vi "calculate tiling positions.vi"(7 "Single Plane?":bool, 8 "error in (no error)":errorcluster, 9 "overlap percentage":dbl) -> (0 "error out 2":errorcluster, 2 "Array 2 - for Zstack tiling use this":dbl[][][](array[numeric]), 3 "2D Array for single plane tiling or Slow Z Tiling":dbl[][](array[numeric]))   [LabVIEW 2012]
doc: "SciScan 1.2 160622"
uses:
  GFG/GFGnumericGet.vi
  GFG/GFGbooleanGet.vi
  GFG/GFG library.lvlib
panel:
  out "Array":dbl[][](array[numeric])
  out "error out":errorcluster
  out "data":dbl[][](array[numeric])
  out "3D Array for Standard Z Tiling":dbl[][][](array[numeric])
  in  "no of frames per tile":dbl
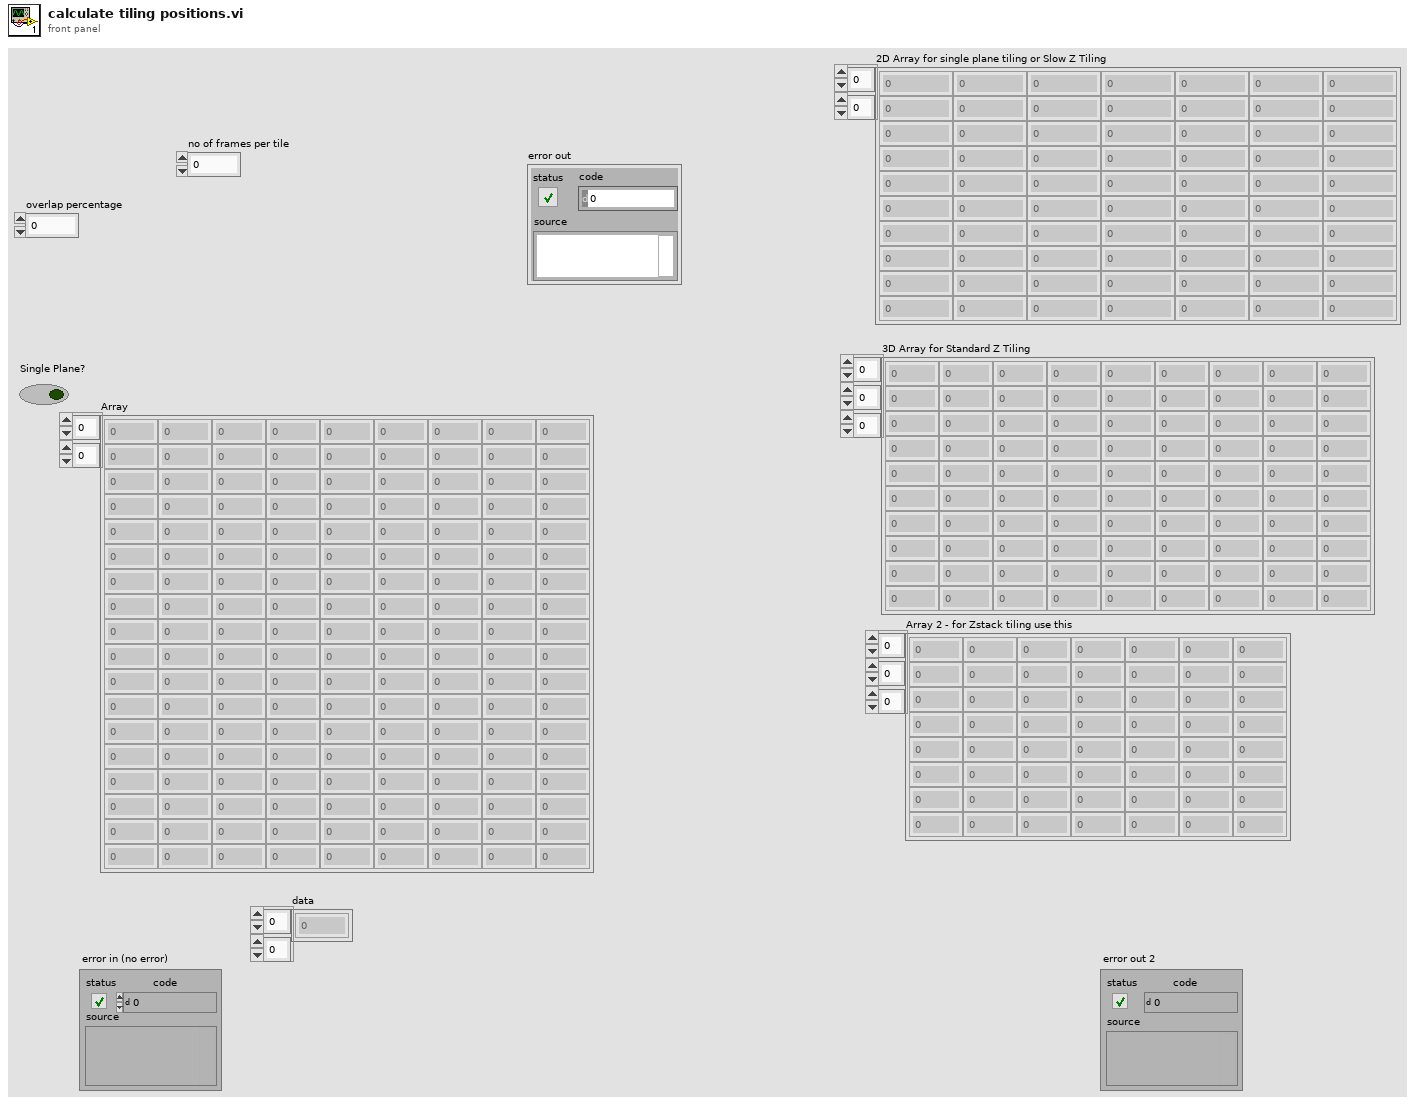
[diagram p1: front panel]
types:
  T1 = cluster{"moveXabs":dbl, "moveYabs":dbl, "moveZabs":dbl}
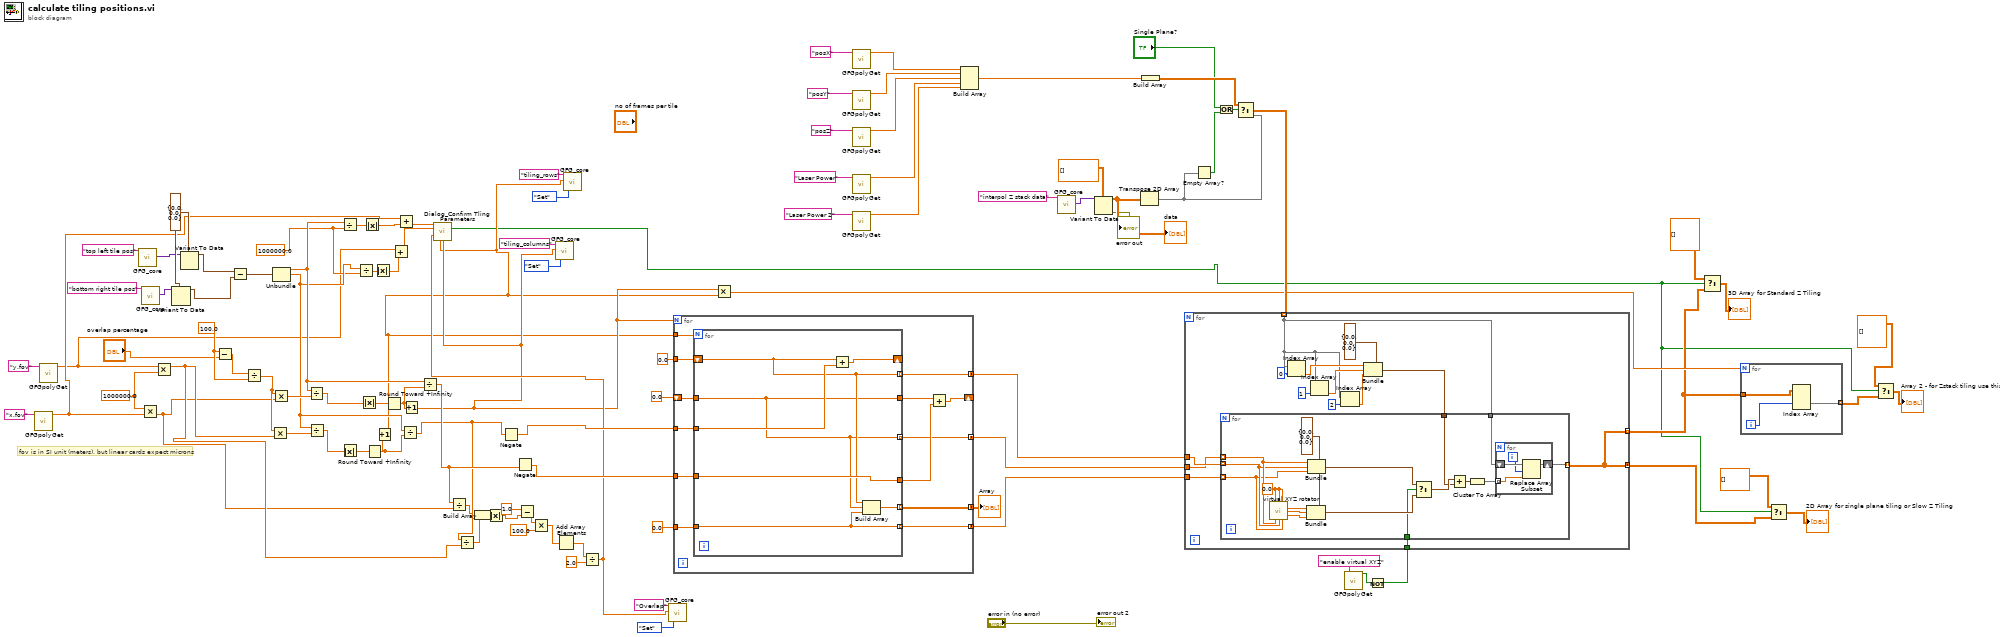
[diagram p0: block diagram]
diagram:
  w22 = 1000000.0 ("y")
  w51 = 1000000.0 ("y")
  w67 = cluster{"rel x":dbl, "rel y":dbl, "rel z":dbl} {"rel x"=0.0, "rel y"=0.0, "rel z"=0.0} ("top left")
  w55 = 100.0 ("x")
  # "fov is in SI unit (meters), but linear cards expect microns"
  n1 = call-poly "GFGpolyGet.vi"("Variable Name in"="x.fov") -> ("Numeric"=w4:dbl)  [unwired: 8 in, 2 out]
  n2 = call-poly "GFGpolyGet.vi"("Variable Name in"="y.fov") -> ("Numeric"=w3:dbl)  [unwired: 8 in, 2 out]
  n3 = call "GFG_core.vi"("Variable Name in"="top left tile pos") -> ("Variant Out"=w63:variant)  [unwired: 12 in, 6 out]
  n4 = call "GFG_core.vi"("Variable Name in"="bottom right tile pos") -> ("Variant Out"=w65:variant)  [unwired: 12 in, 6 out]
  n5 = Multiply(x=w51, y=w4) -> (x*y=w26:dbl)
  n6 = Multiply(x=w3, y=w51) -> (x*y=w27:dbl)
  n7 = Variant To Data(type=w67, Variant=w65) -> (data=w66:cluster{"rel x":dbl, "rel y":dbl, "rel z":dbl})  [unwired: 1 in, 1 out]
  n8 = Variant To Data(type=w67, Variant=w63) -> (data=w64:cluster{"rel x":dbl, "rel y":dbl, "rel z":dbl})  [unwired: 1 in, 1 out]
  n9 = Subtract(x=w55, y="overlap percentage") -> (x-y=w54:dbl)
  n10 = Subtract(x=w64, y=w66) -> (x-y=w53:cluster{"rel x":dbl, "rel y":dbl, "rel z":dbl})
  n11 = Divide(x=w54, y=w55) -> (x/y=w50:dbl)
  n12 = Multiply(x=w50, y=w27) -> (x*y=w56:dbl)
  n13 = Unbundle(w53) -> ("rel x"=w24:dbl, "rel y"=w23:dbl)  [unwired: 1 out]
  n14 = Multiply(x=w50, y=w26) -> (x*y=w57:dbl)
  n15 = Divide(x=w24, y=w57) -> (x/y=w60:dbl)
  n16 = Divide(x=w23, y=w56) -> (x/y=w49:dbl)
  n17 = Divide(x=w24, y=w22) -> (x/y=w21:dbl)
  n18 = Absolute Value(x=w49) -> (abs(x)=w58:dbl)
  n19 = Divide(x=w23, y=w22) -> (x/y=w20:dbl)
  n20 = Absolute Value(x=w60) -> (abs(x)=w59:dbl)
  n21 = Absolute Value(x=w21) -> (abs(x)=w2:dbl)
  n22 = Round Toward +Infinity(x=w58) -> (ceil(x): smallest int >= x=w43:dbl)
  n23 = Absolute Value(x=w20) -> (abs(x)=w1:dbl)
  n24 = Increment(x=w43) -> (x+1=w17:dbl)
  n25 = Round Toward +Infinity(x=w59) -> (ceil(x): smallest int >= x=w44:dbl)
  n26 = Add(x=w3, y=w1) -> (x+y=w5:dbl)
  n27 = Add(x=w4, y=w2) -> (x+y=w6:dbl)
  n28 = Divide(x=w23, y=w43) -> (x/y=w37:dbl)
  n29 = Increment(x=w44) -> (x+1=w18:dbl)
  n30 = Divide(x=w24, y=w44) -> (x/y=w38:dbl)
  n31 = Divide(x=w38, y=w26) -> (x/y=w36:dbl)
  n32 = Divide(x=w37, y=w27) -> (x/y=w35:dbl)
  n33 = Build Array(w36, w35) -> (w33:dbl[])
  n34 = Absolute Value(x=w33) -> (abs(x)=w25:dbl[])
  n35 = Negate(x=w37) -> (-x=w42:dbl)
  n36 = Negate(x=w38) -> (-x=w41:dbl)
  n37 = Subtract(x=1.0, y=w25) -> (x-y=w32:dbl[])
  n38 = Multiply(x=w32, y=100.0 ("x")) -> (x*y=w30:dbl[])
  n39 = call "GFG_core.vi"("Variable Name in"="tiling_columns", "Variant in"=w18, "Action"=enum16{"Init", "Set", "Get", "Clear"}."Set") -> ()  [unwired: 10 in, 7 out]
  n40 = Add Array Elements(numeric array=w30) -> (sum=w29:dbl)
  n41 = call "GFG_core.vi"("Variable Name in"="tiling_rows", "Variant in"=w17, "Action"=enum16{"Init", "Set", "Get", "Clear"}."Set") -> ()  [unwired: 10 in, 7 out]
  n42 = Divide(x=w29, y=2.0) -> (x/y=w19:dbl)
  n43 = call "Dialog_Confirm Tling Parameters.vi"("x FOV"=w6, "y FOV"=w5, "actual \noverlap\npercentage"=w19, "Tiling Rows"=w17, "Tiling Columns"=w18) -> ("Cancelled?"=w7:bool)  [unwired: 9 in, 1 out]
  n44 = call "GFG_core.vi"("Variable Name in"="Overlap", "Variant in"=w19, "Action"=enum16{"Init", "Set", "Get", "Clear"}."Set") -> ()  [unwired: 10 in, 7 out]
  n45 = for {
    N: w18 -> [_]
    shift-right: [w113] -> _
    shift-left: 0.0 ("Numeric") -> [w115]
    tunnel: w42 -> [w112]
    tunnel: [w111] -> w98 mode=concatenating
    tunnel: w41 -> [w109]
    tunnel: [w108] -> w97 mode=concatenating
    tunnel: [w107] -> w96 mode=concatenating
    tunnel: w17 -> [w106]
    tunnel: 0.0 ("Numeric") -> [w116]
    tunnel: 0.0 ("Numeric") -> [w105]
    tunnel: [w104] -> w73 mode=concatenating
    n46 = for {
      N: w106 -> [_]
      shift-right: [w122] -> _
      shift-left: w116 -> [w120]
      tunnel: w112 -> [w123]
      tunnel: [w120] -> w111 mode=indexing
      tunnel: [w121] -> w110
      tunnel: w109 -> [w121]
      tunnel: [w119] -> w108 mode=indexing
      tunnel: w105 -> [w118]
      tunnel: [w118] -> w107 mode=indexing
      tunnel: w115 -> [w119]
      tunnel: [w119] -> w114
      tunnel: [w117] -> w104 mode=indexing
      n47 = Add(x=w120, y=w123) -> (x+y=w122:dbl)
      n48 = Build Array(w120, w119, w118) -> (w117:dbl[])
    }
    n49 = Add(x=w114, y=w110) -> (x+y=w113:dbl)
  }
  "Array" <- w73
  n50 = Multiply(x=w18, y=w17) -> (x*y=w72:dbl)
  n51 = call-poly "GFGpolyGet.vi"("Variable Name in"="posX") -> ("Numeric"=w84:dbl)  [unwired: 8 in, 2 out]
  n52 = call-poly "GFGpolyGet.vi"("Variable Name in"="posY") -> ("Numeric"=w85:dbl)  [unwired: 8 in, 2 out]
  n53 = call-poly "GFGpolyGet.vi"("Variable Name in"="posZ") -> ("Numeric"=w86:dbl)  [unwired: 8 in, 2 out]
  n54 = call-poly "GFGpolyGet.vi"("Variable Name in"="Laser Power") -> ("Numeric"=w87:dbl)  [unwired: 8 in, 2 out]
  n55 = call-poly "GFGpolyGet.vi"("Variable Name in"="Laser Power 2") -> ("Numeric"=w88:dbl)  [unwired: 8 in, 2 out]
  n56 = Build Array(w84, w85, w86, w87, w88) -> (w77:dbl[])
  n57 = call "GFG_core.vi"("Variable Name in"="interpol Z stack data") -> ("Variant Out"=w92:variant)  [unwired: 12 in, 6 out]
  n58 = Variant To Data(type=dbl[][] [], Variant=w92) -> (data=w90:dbl[][], error out=→"error out":errorcluster)  [unwired: 1 in]
  "data" <- w90
  n59 = Transpose 2D Array(2D array=w90) -> (transposed array=w75:dbl[][])
  n60 = Build Array(w77) -> (w76:dbl[][])
  n61 = Empty Array?(array=w75) -> (empty?=w70:bool)
  n62 = Or(x="Single Plane?", y=w70) -> (x .or. y?=w68:bool)
  n63 = Select(t=w76, s=w68, f=w75) -> (s? t:f=w78:dbl[][])
  n64 = call-poly "GFGpolyGet.vi"("Variable Name in"="enable virtual XYZ") -> ("Boolean Value OUT"=w100:bool)  [unwired: 9 in, 1 out]
  n65 = Not(x=w100) -> (.not. x?=w99:bool)
  n66 = for {
    tunnel: w99 -> [w137]
    tunnel: w98 -> [w125]
    tunnel: w97 -> [w124]
    tunnel: w96 -> [w136]
    tunnel: w78 -> [w127] mode=indexing
    tunnel: [w126] -> w16 mode=concatenating
    tunnel: [w126] -> w10 mode=indexing
    n67 = Index Array(array=w127, index=0) -> (element=w134:dbl)
    n68 = Index Array(array=w127, index=1) -> (element=w133:dbl)
    n69 = Index Array(array=w127, index=2) -> (element=w130:dbl)
    n70 = Bundle(cluster=T1 {"moveXabs"=0.0, "moveYabs"=0.0, "moveZabs"=0.0} ("output cluster"), "moveXabs"=w134, "moveYabs"=w133, "moveZabs"=w130) -> (w128:T1)
    n71 = for {
      tunnel: w137 -> [w148]
      tunnel: w128 -> [w145]
      tunnel: w124 -> [w144] mode=indexing
      tunnel: w125 -> [w143] mode=indexing
      tunnel: w136 -> [w142] mode=indexing
      tunnel: [w138] -> w126 mode=indexing
      tunnel: w127 -> [w140]
      w147 = 0.0 ("current pos X")
      w151 = T1 {"moveXabs"=0.0, "moveYabs"=0.0, "moveZabs"=0.0} ("output cluster")
      n72 = call "virtual XYZ rotator.vi"("current pos X"=w147, "current pos Y"=w147, "current pos Z"=w147, "virtual X relative"=w144, "virtual Y relative"=w143, "virtual Z relative"=w142) -> ("new pos X"=w154:dbl, "new pos Y"=w153:dbl, "new pos Z"=w152:dbl)  [unwired: 7 in]
      n73 = Bundle(cluster=w151, "moveXabs"=w154, "moveYabs"=w153, "moveZabs"=w152) -> (w149:T1)
      n74 = Bundle(cluster=w151, "moveXabs"=w144, "moveYabs"=w143, "moveZabs"=w142) -> (w150:T1)
      n75 = Select(t=w150, s=w148, f=w149) -> (s? t:f=w146:T1)
      n76 = Add(x=w146, y=w145) -> (x+y=w141:T1)
      n77 = Cluster To Array(cluster=w141) -> (array=w139:dbl[])
      n78 = for {
        shift-right: [w157] -> w138
        shift-left: w140 -> [w158]
        tunnel: w139 -> [w155] mode=indexing
        i -> [w156]
        n79 = Replace Array Subset(array=w158, new element=w155, index=w156) -> (w157:dbl[])
      }
    }
  }
  n80 = Select(t=dbl[][][] [], s=w7, f=w10) -> (s? t:f=→"3D Array for Standard Z Tiling":dbl[][][])
  n81 = for {
    N: w72 -> [_]
    tunnel: [w161] -> w13 mode=indexing
    tunnel: w10 -> [w160]
    i -> [w159]
    n82 = Index Array(array=w160, index (dim 1)=w159) -> (element=w161:dbl[][])  [unwired: 2 in]
  }
  n83 = Select(t=dbl[][] [], s=w7, f=w16) -> (s? t:f=→"2D Array for single plane tiling or Slow Z Tiling":dbl[][])
  n84 = Select(t=dbl[][][] [], s=w7, f=w13) -> (s? t:f=→"Array 2 - for Zstack tiling use this":dbl[][][])
  "error out 2" <- "error in (no error)"
